vi "gmail.vi"() -> ()   [LabVIEW 2019]
panel:
  in  "CC (Carbon Copy Recipient - Optional)":string
  in  "Recipient's Email Address Address":string
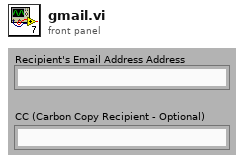
[diagram p1: front panel]
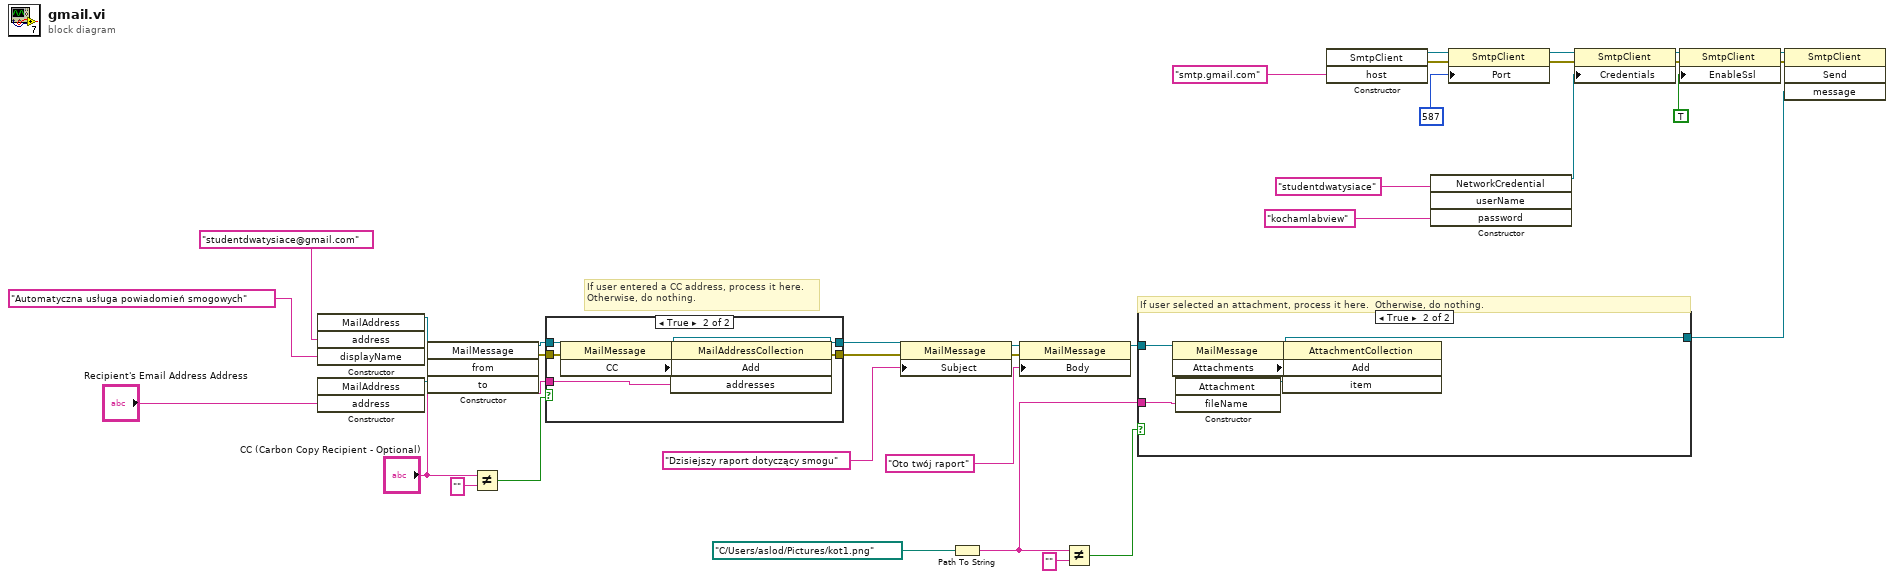
[diagram p0: block diagram]
diagram:
  # "If user selected an attachment, process it here.  Otherwise, do nothing."
  # "If user entered a CC address, process it here.\nOtherwise, do nothing."
  n1 = constructor class="MailAddress"("address"="studentdwatysiace@gmail.com" ("Sender's Email Address (eg: jsmith77@gmail.com)"), "displayName"="Automatyczna usługa powiadomień smogowych" ("Sender's Name")) -> (reference out=w35:refnum<k24>)  [unwired: 3 in, 4 out]
  n2 = constructor class="MailAddress"("address"="Recipient's Email Address Address") -> (reference out=w36:refnum<k24>)  [unwired: 3 in, 3 out]
  n3 = constructor class="MailMessage"("from"=w35, "to"=w36) -> (reference out=w5:refnum<k24>, error out=w4:errorcluster)  [unwired: 3 in, 3 out]
  n4 = Not Equal?(x="CC (Carbon Copy Recipient - Optional)", y="") -> (x != y?=w7:bool)
  n5 = case shown="True" w7 {
    tunnel: "CC (Carbon Copy Recipient - Optional)" -> [_ w43]
    tunnel: w5 -> [w38 w42]
    tunnel: w4 -> [w37 w41]
    tunnel: [w38 w40] -> w3
    tunnel: [w37 w39] -> w2
    frame False {
    }
    frame True {
      n6 = property class="MailMessage"(reference=w42, error in=w41) -> (reference out=w40:refnum<k24>, error out=w45:errorcluster, "CC"=w44:refnum<k24>)
      n7 = invoke class="MailAddressCollection" method="Add"(reference=w44, error in=w45, "addresses"=w43) -> (error out=w39:errorcluster)  [unwired: 1 in, 3 out]
    }
  }
  n8 = property class="MailMessage"(reference=w3, error in=w2, "Subject"="Dzisiejszy raport dotyczący smogu") -> (reference out=w28:refnum<k24>, error out=w34:errorcluster)
  n9 = Path To String(path=path "C:/Users/aslod/Pictures/kot1.png" ("Attachment - Optional")) -> (string=w9:string)
  n10 = property class="MailMessage"(reference=w28, error in=w34, "Body"="Oto twój raport") -> (reference out=w14:refnum<k24>)  [unwired: 1 out]
  n11 = Not Equal?(x=w9, y="") -> (x != y?=w10:bool)
  n12 = case shown="True" w10 {
    tunnel: w14 -> [w46 w49]
    tunnel: [w46 w48] -> w13
    tunnel: w9 -> [_ w47]
    frame False {
    }
    frame True {
      n13 = property class="MailMessage"(reference=w49) -> (reference out=w48:refnum<k24>, error out=w52:errorcluster, "Attachments"=w50:refnum<k24>)  [unwired: 1 in]
      n14 = constructor class="Attachment"("fileName"=w47) -> (reference out=w51:refnum<k24>)  [unwired: 3 in, 3 out]
      n15 = invoke class="AttachmentCollection" method="Add"(reference=w50, error in=w52, "item"=w51) -> ()  [unwired: 1 in, 4 out]
    }
  }
  n16 = constructor class="SmtpClient"("host"="smtp.gmail.com" ("Outgoing Mail Server (SMTP)")) -> (reference out=w22:refnum<k24>, error out=w18:errorcluster)  [unwired: 3 in, 2 out]
  n17 = constructor class="NetworkCredential"("userName"="studentdwatysiace" ("GMAIL Account User ID (eg: jsmity77)"), "password"="kochamlabview" ("GMAIL Account Password")) -> (reference out=w23:refnum<k24>)  [unwired: 3 in, 4 out]
  n18 = property class="SmtpClient"(reference=w22, error in=w18, "Port"=587) -> (reference out=w21:refnum<k24>, error out=w17:errorcluster)
  n19 = property class="SmtpClient"(reference=w21, error in=w17, "Credentials"=w23) -> (reference out=w20:refnum<k24>, error out=w16:errorcluster)
  n20 = property class="SmtpClient"(reference=w20, error in=w16, "EnableSsl"=TRUE ("Enable SSL")) -> (reference out=w19:refnum<k24>, error out=w15:errorcluster)
  n21 = invoke class="SmtpClient" method="Send"(reference=w19, error in=w15, "message"=w13) -> ()  [unwired: 1 in, 4 out]
